vi "Adjust Pixel Overlay Brightness.vi"(5 "Scale Max":dbl, 7 "Scale Min":dbl, 8 "Error In":errorcluster, 9 "Pixel in":sgl, 10 "Pixel Color Value (black)":T1, 11 "Overlay Color Value in":T1) -> (0 "Error Out":errorcluster, 3 "Overlay Color Value out":T1)   [LabVIEW 2021, in "Image.lvlib"]
doc: "Scales the brightness of a RGB <B>Overlay Volor Value in</B> according to the value of <B>Pixel in</B> and <B>Scale Min</B> & <B>Scale Max</B> according to:\n\nR,G,B out = R,G,B in x f\nf = (Pixel in - Scale Min)/(Scale Max - Scale Min)\n\nwhere a value of 0 is used for f if Pixel in < Scale Min and a value of 1 if Pixel in > Scale Max.\n\nIf <B>Pixel Color Value</B> is provided, the overlay color is blended with that of the pixel such that for a <B>Pixel in</B> value of <B>Scale Min</B>, the overlay color is identical to that of the pixel:\n\nR,G,B out = R,G,B in x f + Pixel Color in x (1 - f)\nf = (Pixel in - Scale Min)/(Scale Max - Scale Min)"
uses:
  Image.lvlib
  Comparison/Comparison.lvlib
panel:
  # "see the AlliGator License on the block diagram (Ctrl+E or Window:Show Block Diagram)"
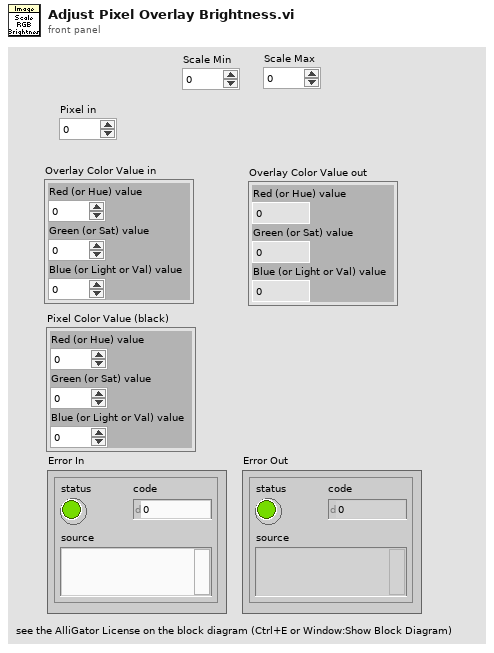
[diagram p1: front panel]
types:
  T1 = cluster{"Red (or Hue) value":u8, "Green (or Sat) value":u8, "Blue (or Light or Val) value":u8}
  T2 = cluster{"Red (or Hue) value":bool, "Green (or Sat) value":bool, "Blue (or Light or Val) value":bool}
  T3 = cluster{"Red (or Hue) value":dbl, "Green (or Sat) value":dbl, "Blue (or Light or Val) value":dbl}
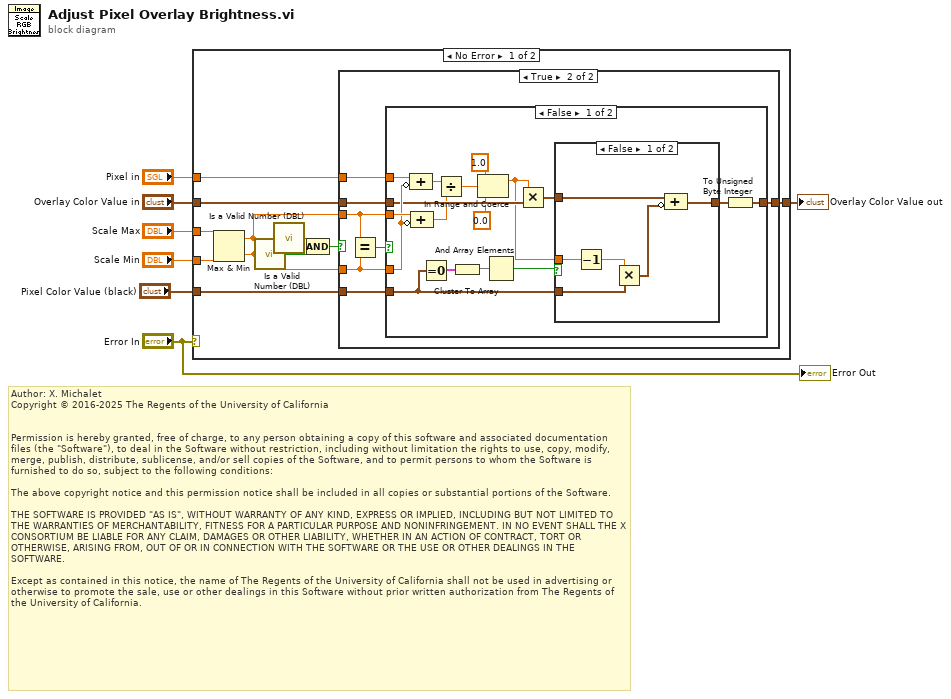
[diagram p0: block diagram]
diagram:
  # "Author: X. Michalet\nCopyright © 2016-2025 The Regents of the University of California\n \n\nPermission is hereby granted, free of charge, to any person obtaining a copy of this software and associated documentation files (the \"Software\"), to deal in the Software without restriction, including without limitation the rights to use, copy, modify, merge, publish, distribute, sublicense, and/or sell copies of the Software, and to permit persons to whom the Software is furnished to do so, subject to the following conditions:\n\nThe above copyright notice and this permission notice shall be included in all copies or substantial portions of the Software.\n\nTHE SOFTWARE IS PROVIDED \"AS IS\", WITHOUT WARRANTY OF ANY KIND, EXPRESS OR IMPLIED, INCLUDING BUT NOT LIMITED TO THE WARRANTIES OF MERCHANTABILITY, FITNESS FOR A PARTICULAR PURPOSE AND NONINFRINGEMENT. IN NO EVENT SHALL THE X CONSORTIUM BE LIABLE FOR ANY CLAIM, DAMAGES OR OTHER LIABILITY, WHETHER IN AN ACTION OF CONTRACT, TORT OR OTHERWISE, ARISING FROM, OUT OF OR IN CONNECTION WITH THE SOFTWARE OR THE USE OR OTHER DEALINGS IN THE SOFTWARE.\n\nExcept as contained in this notice, the name of The Regents of the University of California shall not be used in advertising or otherwise to promote the sale, use or other dealings in this Software without prior written authorization from The Regents of the University of California."
  n1 = case shown="No Error" "Error In" {
    tunnel: "Pixel in" -> [w18 _]
    tunnel: "Scale Max" -> [w14 _]
    tunnel: "Scale Min" -> [w13 _]
    tunnel: "Overlay Color Value in" -> [w10 w52]
    tunnel: [w9 w52] -> w2
    tunnel: "Pixel Color Value (black)" -> [w8 _]
    frame No Error {
      n2 = Max & Min(x=w14, y=w13) -> (max(x,y)=w12:dbl, min(x,y)=w11:dbl)
      n3 = call "Is a Valid Number (DBL).vi"("Number"=w11) -> ("Valid Number?"=w16:bool)  [unwired: 8 in]
      n4 = call "Is a Valid Number (DBL).vi"("Number"=w12) -> ("Valid Number?"=w17:bool)  [unwired: 8 in]
      n5 = Compound Arithmetic op=AND(w17, w16) -> (w15:bool)
      n6 = case shown="True" w15 {
        tunnel: w18 -> [_ w26]
        tunnel: w11 -> [_ w22]
        tunnel: w12 -> [_ w21]
        tunnel: w10 -> [w19 w24]
        tunnel: [w19 w23] -> w9
        tunnel: w8 -> [_ w20]
        frame False {
          # "If scale min or max are Inf or NaN, do nothing"
        }
        frame True {
          n7 = Equal?(x=w21, y=w22) -> (x = y?=w25:bool)
          n8 = case shown="False" w25 {
            tunnel: w26 -> [w43 _]
            tunnel: w24 -> [w40 w51]
            tunnel: [w33 w51] -> w23
            tunnel: w22 -> [w41 _]
            tunnel: w21 -> [w42 _]
            tunnel: w20 -> [w30 _]
            frame False {
              n9 = Compound Arithmetic op=ADD(w43, invert w41) -> (w38:dbl)
              n10 = Compound Arithmetic op=ADD(w42, invert w41) -> (w37:dbl)
              n11 = Equal To 0?(x=w30) -> (x = 0?=w29:T2)
              n12 = Divide(x=w38, y=w37) -> (x/y=w36:dbl)
              n13 = Cluster To Array(cluster=w29) -> (array=w28:bool[])
              n14 = In Range and Coerce(upper limit=1.0, x=w36, lower limit=0.0) -> (coerced(x)=w32:dbl)  [unwired: 1 out]
              n15 = And Array Elements(Boolean array=w28) -> (logical AND=w27:bool)
              n16 = Multiply(x=w32, y=w40) -> (x*y=w39:T3)
              n17 = case shown="False" w27 {
                tunnel: w39 -> [w49 w50]
                tunnel: w30 -> [w48 _]
                tunnel: w32 -> [w47 _]
                tunnel: [w45 w50] -> w31
                frame False {
                  n18 = Decrement(x=w47) -> (x-1=w46:dbl)
                  n19 = Multiply(x=w46, y=w48) -> (x*y=w44:T3)
                  n20 = Compound Arithmetic op=ADD(w49, invert w44) -> (w45:T3)
                }
                frame True {
                  # "if black pixel, skip"
                }
              }
              n21 = To Unsigned Byte Integer(number=w31) -> (unsigned 8bit integer=w33:T1)
            }
            frame True {
              # "if the scale min = max, then do nothing"
            }
          }
        }
      }
    }
    frame Error {
    }
  }
  "Overlay Color Value out" <- w2
  "Error Out" <- "Error In"
